vi "Get Type.vi"(0 "video writer in":refnum<class "MSC Video Writer.lvclass">, 5 "error in (no error)":errorcluster) -> (14 "video writer out":refnum<class "MSC Video Writer.lvclass">, 15 "Type":T1 items=["Grayscale U8"=0, "Grayscale U16"=2, "Grayscale Single"=5, "Grayscale Double"=6, "RGB U8"=16], 19 "error out":errorcluster)   [LabVIEW 2014, in "MSC Video Writer.lvclass"]
doc: "Reads the type of the video."
uses:
  MSC Video Writer.lvclass
  MSC Image_class/controls/Image Type.ctl
  MSC Video Writer.lvclass/MSC Video Writer.ctl
  MSC Image_class/MSC Image.lvclass
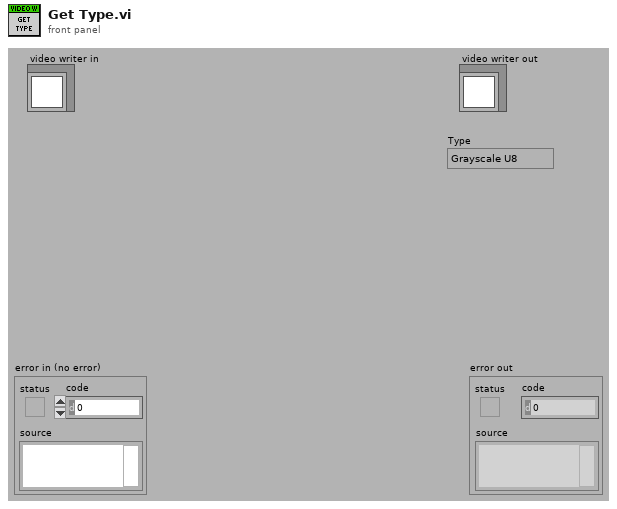
[diagram p1: front panel]
types:
  T1 = typedef "MSC Image.lvclass/Image Type.ctl" = i32
  T2 = typedef "MSC Video Writer.lvclass/Video Writer.ctl" = cluster{"Pointer":u64, "FPS":u32, "Path":path, "FourCC Codec":string, "Size":T3, "Type":T1}
  T3 = typedef "MSC Image.lvclass/Size.ctl" = cluster{"Cols":i32, "Rows":i32}
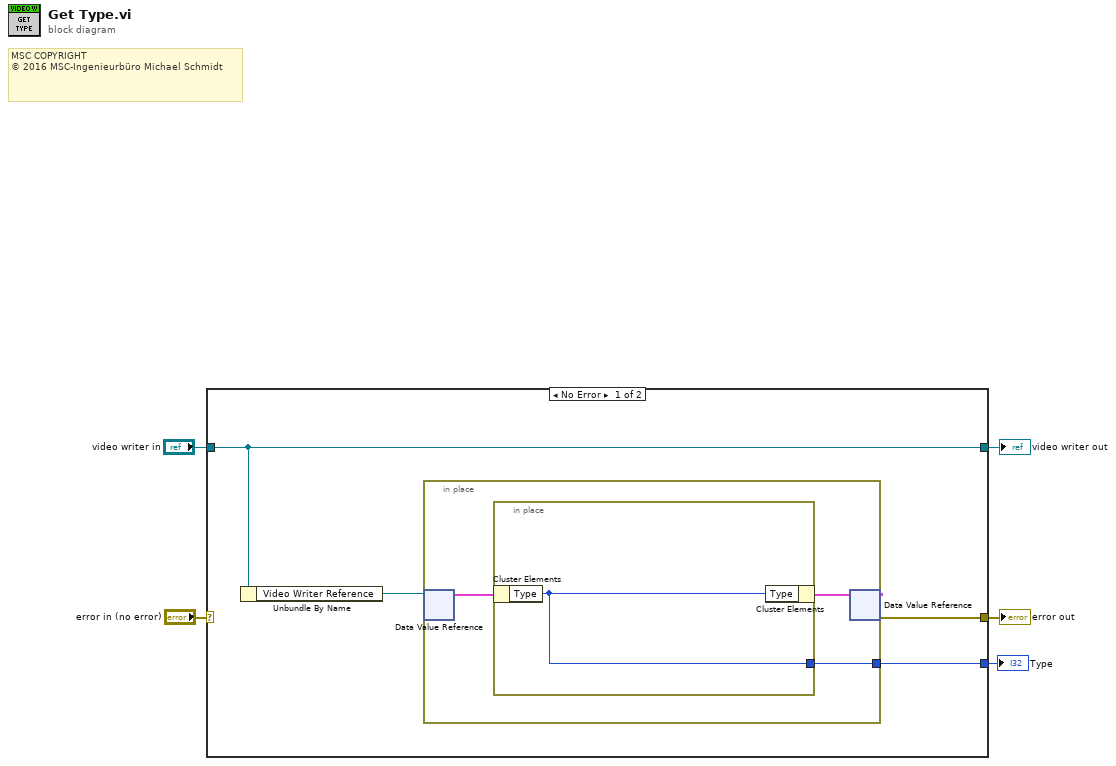
[diagram p0: block diagram]
diagram:
  # "MSC COPYRIGHT\n© 2016 MSC-Ingenieurbüro Michael Schmidt"
  # "MSC COPYRIGHT\n© 2016 MSC-Ingenieurbüro Michael Schmidt"
  n1 = case shown="No Error" "error in (no error)" {
    selector: "error in (no error)" -> [_ w15]
    tunnel: [w8 w15] -> w4
    tunnel: [w9 w14] -> w2
    tunnel: "video writer in" -> [w9 w14]
    tunnel: [w6 _] -> w1
    frame No Error {
      n2 = Unbundle By Name(w9) -> ("Video Writer Reference"=w7:refnum<data-value>)
      n3 = in-place {
        in-place-border: [w10] -> w6
        n4 = in-place-dvr #1(w7) -> (w11:T2)  [unwired: 1 out]
        n5 = in-place {
          in-place-border: [w13] -> w10
          n6 = in-place-cluster #2(w11) -> ("Type"=w13:T1)
          n7 = in-place-cluster #2("Type"=w13) -> (w12:T2)
        }
        n8 = in-place-dvr #1(w12) -> (w8:errorcluster)  [unwired: 1 out]
      }
    }
    frame Error {
    }
  }
  "error out" <- w4
  "video writer out" <- w2
  "Type" <- w1
